vi "Círculo de Mohr Excel.vi"(0 "Array in":cluster{"Array":dbl[], "Array":dbl[]}[](array[cluster])) -> (1 "Array out":dbl[][](array[numeric]), 2 "Cluster 2":T1, 3 "Cluster":T1)   [LabVIEW 2013]
uses:
  <vilib>/gmath/NI_Gmath.lvlib
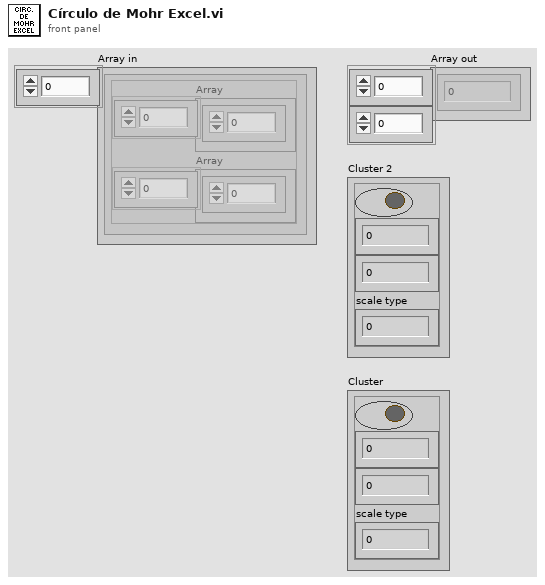
[diagram p1: front panel]
types:
  T1 = cluster{"Boolean":bool, "Numeric Control":dbl, "Numeric Control":dbl, "scale type":i32}
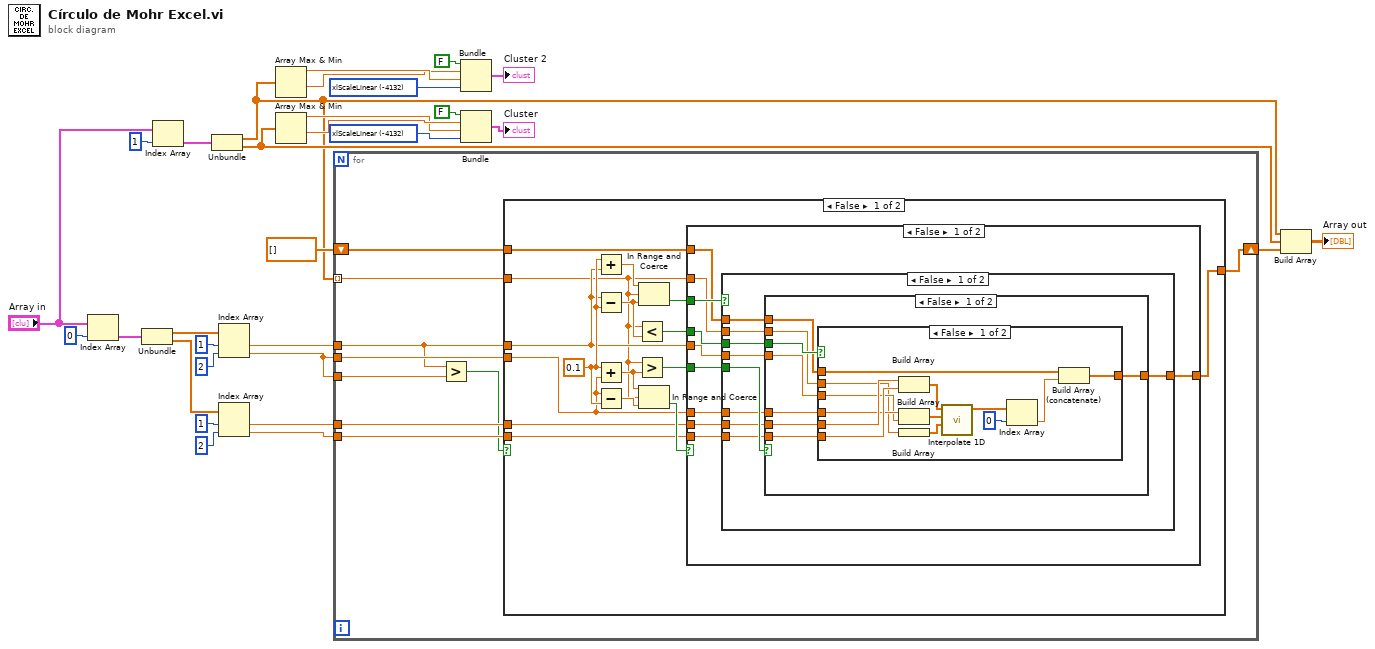
[diagram p0: block diagram]
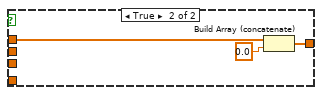
[diagram p2: hidden frame]
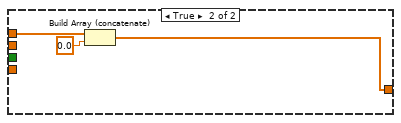
[diagram p3: hidden frame]
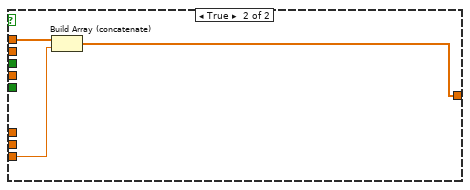
[diagram p4: hidden frame]
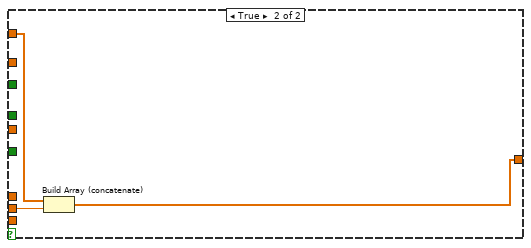
[diagram p5: hidden frame]
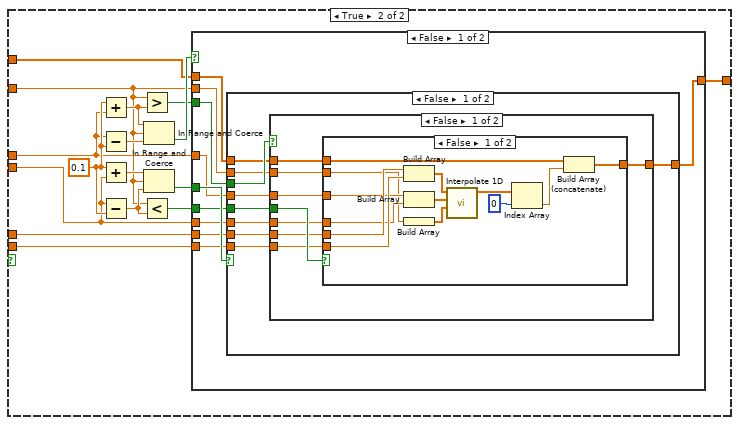
[diagram p6: hidden frame]
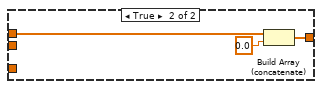
[diagram p7: hidden frame]
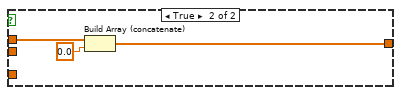
[diagram p8: hidden frame]
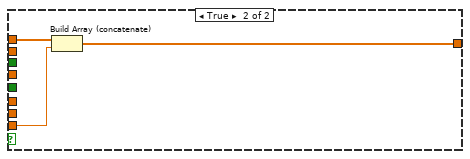
[diagram p9: hidden frame]
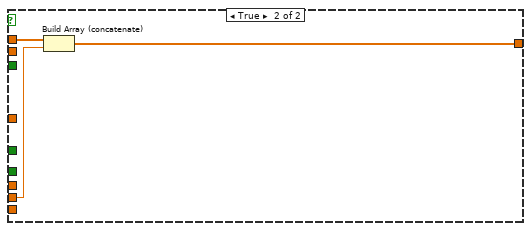
[diagram p10: hidden frame]
diagram:
  w26 = -4132 items=["xlScaleLinear"=-4132, "xlScaleLogarithmic"=-4133] ("scale type")
  w24 = -4132 items=["xlScaleLinear"=-4132, "xlScaleLogarithmic"=-4133] ("scale type")
  n1 = Index Array(array="Array in", index=0) -> (element=w14:cluster{"Array":dbl[], "Array":dbl[]})
  n2 = Unbundle(w14) -> ("Array"=w13:dbl[], "Array"=w7:dbl[])
  n3 = Index Array(array="Array in", index=1) -> (element=w20:cluster{"Array":dbl[], "Array":dbl[]})
  n4 = Unbundle(w20) -> ("Array"=w3:dbl[], "Array"=w17:dbl[])
  n5 = Index Array(array=w13, index #1=1 ("index"), index #2=2 ("index")) -> (element #1=w10:dbl, element #2=w1:dbl)
  n6 = Index Array(array=w7, index #1=1 ("index"), index #2=2 ("index")) -> (element #1=w6:dbl, element #2=w4:dbl)
  n7 = Array Max & Min(array=w3) -> (max value=w16:dbl, min value=w15:dbl)  [unwired: 2 out]
  n8 = Array Max & Min(array=w17) -> (max value=w28:dbl, min value=w30:dbl)  [unwired: 2 out]
  n9 = for {
    tunnel: w10 -> [w33]
    tunnel: w1 -> [w35]
    tunnel: w3 -> [w34] mode=indexing
    tunnel: w6 -> [w39]
    shift-right: [w38] -> w2
    shift-left: dbl[] [] -> [w37]
    tunnel: w4 -> [w36]
    tunnel: w1 -> [w32]
    n10 = Greater?(x=w33, y=w32) -> (0:w31:bool)
    n11 = case shown="False" w31 {
      tunnel: w39 -> [w41 w117]
      tunnel: [w40 w116] -> w38
      tunnel: w37 -> [w46 w115]
      tunnel: w36 -> [w42 w113]
      tunnel: w35 -> [w44 w110]
      tunnel: w34 -> [w43 w109]
      tunnel: w33 -> [w45 w108]
      frame False {
        w52 = 0.1
        n12 = Add(x=w52, y=w45) -> (x+y=w54:dbl)
        n13 = Subtract(x=w45, y=w52) -> (x-y=w51:dbl)
        n14 = Add(x=w52, y=w44) -> (x+y=w53:dbl)
        n15 = Subtract(x=w44, y=w52) -> (x-y=w55:dbl)
        n16 = Less?(x=w43, y=w51) -> (x < y?=w47:bool)
        n17 = Greater?(x=w43, y=w53) -> (0:w48:bool)
        n18 = In Range and Coerce(upper limit=w54, x=w43, lower limit=w51) -> (In Range?=w49:bool)  [unwired: 1 out]
        n19 = In Range and Coerce(upper limit=w53, x=w43, lower limit=w55) -> (In Range?=w50:bool)  [unwired: 1 out]
        n20 = case shown="False" w50 {
          tunnel: w41 -> [w59 w107]
          tunnel: [w62 w106] -> w40
          tunnel: w46 -> [w64 w105]
          tunnel: w49 -> [w65 _]
          tunnel: w42 -> [w63 _]
          tunnel: w48 -> [w61 _]
          tunnel: w47 -> [w60 _]
          tunnel: w44 -> [w58 _]
          tunnel: w45 -> [w57 _]
          tunnel: w43 -> [w56 _]
          frame False {
            n21 = case shown="False" w65 {
              tunnel: w64 -> [w73 w104]
              tunnel: w63 -> [w69 w103]
              tunnel: [w72 w102] -> w62
              tunnel: w61 -> [w74 _]
              tunnel: w60 -> [w71 _]
              tunnel: w59 -> [w70 _]
              tunnel: w58 -> [w68 _]
              tunnel: w57 -> [w67 _]
              tunnel: w56 -> [w66 _]
              frame False {
                n22 = case shown="False" w74 {
                  tunnel: w73 -> [w81 w101]
                  tunnel: [w80 w99] -> w72
                  tunnel: w71 -> [w82 _]
                  tunnel: w70 -> [w79 _]
                  tunnel: w69 -> [w78 _]
                  tunnel: w68 -> [w77 _]
                  tunnel: w67 -> [w76 _]
                  tunnel: w66 -> [w75 _]
                  frame False {
                    n23 = case shown="False" w82 {
                      tunnel: w81 -> [w84 w98]
                      tunnel: [w83 w96] -> w80
                      tunnel: w79 -> [w95 _]
                      tunnel: w78 -> [w94 _]
                      tunnel: w77 -> [w92 _]
                      tunnel: w76 -> [w91 _]
                      tunnel: w75 -> [w89 _]
                      frame False {
                        n24 = Build Array(w95, w94) -> (w93:dbl[])
                        n25 = Build Array(w92, w91) -> (w90:dbl[])
                        n26 = Build Array(w89) -> (w88:dbl[])
                        n27 = call <vilib>:"Interpolate 1D.vi"("xi"=w88, "X"=w90, "Y"=w93) -> ("yi"=w87:dbl[])  [unwired: 6 in, 2 out]
                        n28 = Index Array(array=w87, index=0) -> (element=w85:dbl)
                        n29 = Build Array (concatenate)(w84, w85) -> (w83:dbl[])
                      }
                      frame True {
                        n30 = Build Array (concatenate)(w98, 0.0) -> (w96:dbl[])
                      }
                    }
                  }
                  frame True {
                    n31 = Build Array (concatenate)(w101, 0.0) -> (w99:dbl[])
                  }
                }
              }
              frame True {
                n32 = Build Array (concatenate)(w104, w103) -> (w102:dbl[])
              }
            }
          }
          frame True {
            n33 = Build Array (concatenate)(w105, w107) -> (w106:dbl[])
          }
        }
      }
      frame True {
        w120 = 0.1
        n34 = Add(x=w120, y=w108) -> (x+y=w121:dbl)
        n35 = Subtract(x=w108, y=w120) -> (x-y=w123:dbl)
        n36 = Add(x=w120, y=w110) -> (x+y=w122:dbl)
        n37 = Subtract(x=w110, y=w120) -> (x-y=w119:dbl)
        n38 = Greater?(x=w109, y=w121) -> (0:w112:bool)
        n39 = Less?(x=w109, y=w119) -> (x < y?=w111:bool)
        n40 = In Range and Coerce(upper limit=w121, x=w109, lower limit=w123) -> (In Range?=w118:bool)  [unwired: 1 out]
        n41 = In Range and Coerce(upper limit=w122, x=w109, lower limit=w119) -> (In Range?=w114:bool)  [unwired: 1 out]
        n42 = case shown="False" w118 {
          tunnel: w117 -> [w127 w175]
          tunnel: [w130 w174] -> w116
          tunnel: w115 -> [w132 w173]
          tunnel: w114 -> [w133 _]
          tunnel: w113 -> [w131 _]
          tunnel: w112 -> [w129 _]
          tunnel: w111 -> [w128 _]
          tunnel: w108 -> [w126 _]
          tunnel: w110 -> [w125 _]
          tunnel: w109 -> [w124 _]
          frame False {
            n43 = case shown="False" w133 {
              tunnel: w132 -> [w141 w172]
              tunnel: w131 -> [w137 w171]
              tunnel: [w140 w170] -> w130
              tunnel: w129 -> [w142 _]
              tunnel: w128 -> [w139 _]
              tunnel: w127 -> [w138 _]
              tunnel: w126 -> [w136 _]
              tunnel: w125 -> [w135 _]
              tunnel: w124 -> [w134 _]
              frame False {
                n44 = case shown="False" w142 {
                  tunnel: w141 -> [w149 w169]
                  tunnel: [w148 w167] -> w140
                  tunnel: w139 -> [w150 _]
                  tunnel: w138 -> [w147 _]
                  tunnel: w137 -> [w146 _]
                  tunnel: w136 -> [w145 _]
                  tunnel: w135 -> [w144 _]
                  tunnel: w134 -> [w143 _]
                  frame False {
                    n45 = case shown="False" w150 {
                      tunnel: w149 -> [w152 w166]
                      tunnel: [w151 w164] -> w148
                      tunnel: w147 -> [w163 _]
                      tunnel: w146 -> [w162 _]
                      tunnel: w145 -> [w160 _]
                      tunnel: w144 -> [w159 _]
                      tunnel: w143 -> [w157 _]
                      frame False {
                        n46 = Build Array(w163, w162) -> (w161:dbl[])
                        n47 = Build Array(w160, w159) -> (w158:dbl[])
                        n48 = Build Array(w157) -> (w156:dbl[])
                        n49 = call <vilib>:"Interpolate 1D.vi"("xi"=w156, "X"=w158, "Y"=w161) -> ("yi"=w155:dbl[])  [unwired: 6 in, 2 out]
                        n50 = Index Array(array=w155, index=0) -> (element=w153:dbl)
                        n51 = Build Array (concatenate)(w152, w153) -> (w151:dbl[])
                      }
                      frame True {
                        n52 = Build Array (concatenate)(w166, 0.0) -> (w164:dbl[])
                      }
                    }
                  }
                  frame True {
                    n53 = Build Array (concatenate)(w169, 0.0) -> (w167:dbl[])
                  }
                }
              }
              frame True {
                n54 = Build Array (concatenate)(w172, w171) -> (w170:dbl[])
              }
            }
          }
          frame True {
            n55 = Build Array (concatenate)(w173, w175) -> (w174:dbl[])
          }
        }
      }
    }
  }
  n56 = Bundle(FALSE, w15, w16, "scale type"=w24) -> (→"Cluster 2":cluster{bool, dbl, dbl, "scale type":i32})  [unwired: 1 in]
  n57 = Bundle(FALSE, w30, w28, "scale type"=w26) -> (→"Cluster":cluster{bool, dbl, dbl, "scale type":i32})  [unwired: 1 in]
  n58 = Build Array(w3, w17, w2) -> (→"Array out":dbl[][])
